vi "dispense test.vi"() -> ()   [LabVIEW 2021]
uses:
  Classes/Controller/Controller.lvclass
  Classes/Controller/Dispenser/Dispenser.lvclass
panel:
  out "current time 3":timestamp
  out "current time 2":timestamp
  out "current time":timestamp
  out "Adjusted Dispensing Time (ms)":dbl
  out "Start time":timestamp
  out "end time":timestamp
  out "Iteration":i32
  in  "Time (ms)":dbl
  out "Dispense on":bool
  out "error out":errorcluster
  in  "error in (no error)":errorcluster
  in  "Pressure (psi)":i16=20
  in  "Dispense":bool
  in  "stop":bool
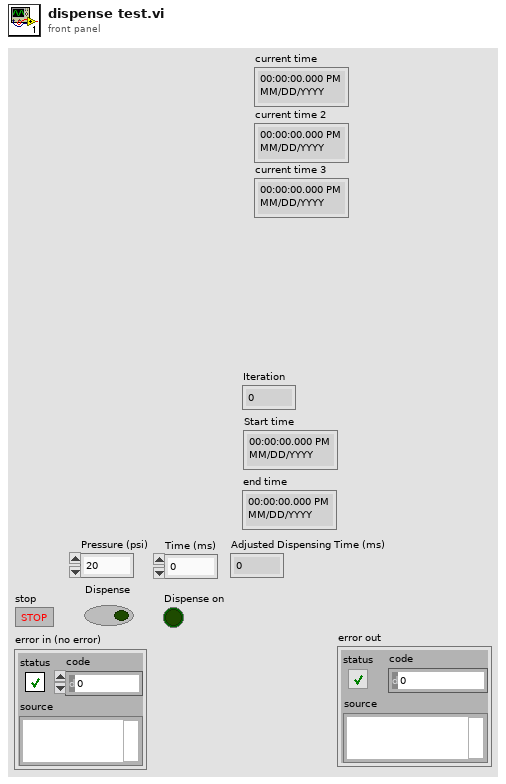
[diagram p1: front panel]
types:
  T1 = typedef "Controller.lvclass/Controllers.ctl" = cluster{"I-O.lvclass":refnum<class "I-O.lvclass">, "Gantry":refnum<k24>, "Dispenser":refnum<visa-resource-name>}
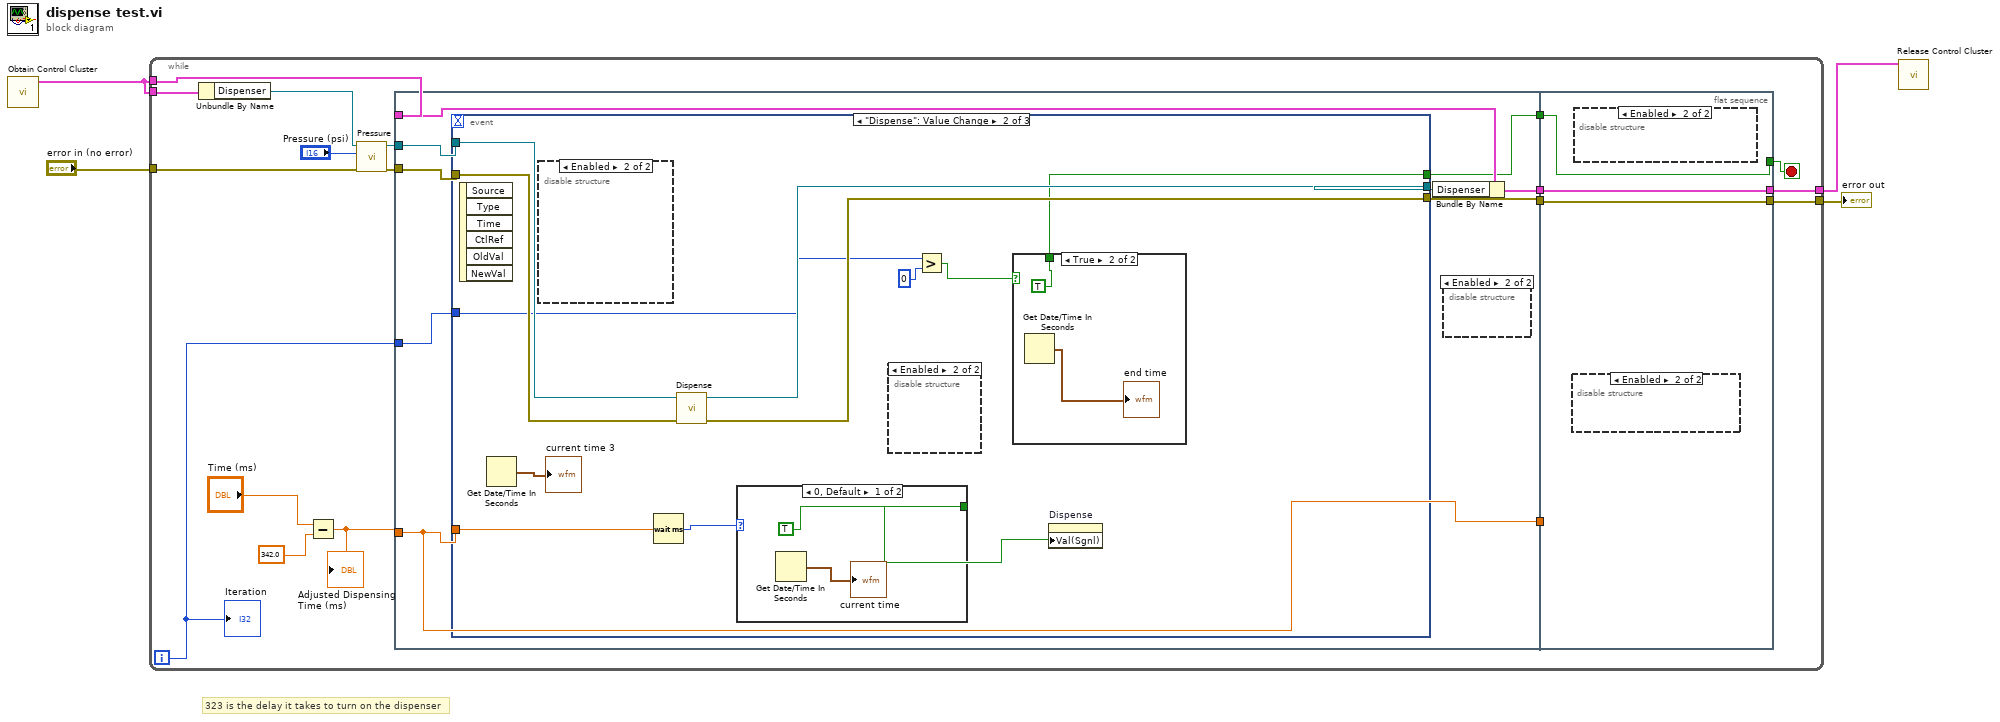
[diagram p0: block diagram]
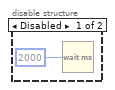
[diagram p2: hidden frame]
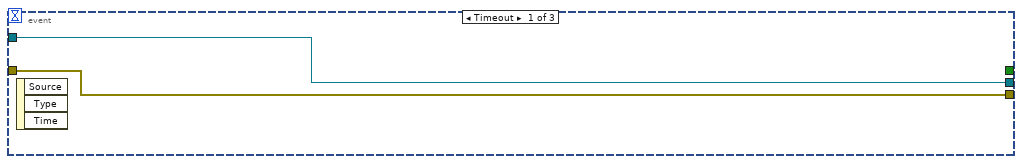
[diagram p3: hidden frame]
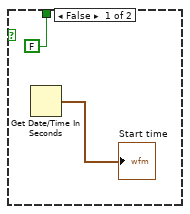
[diagram p4: hidden frame]
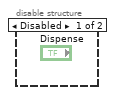
[diagram p5: hidden frame]
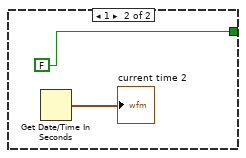
[diagram p6: hidden frame]
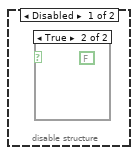
[diagram p7: hidden frame]
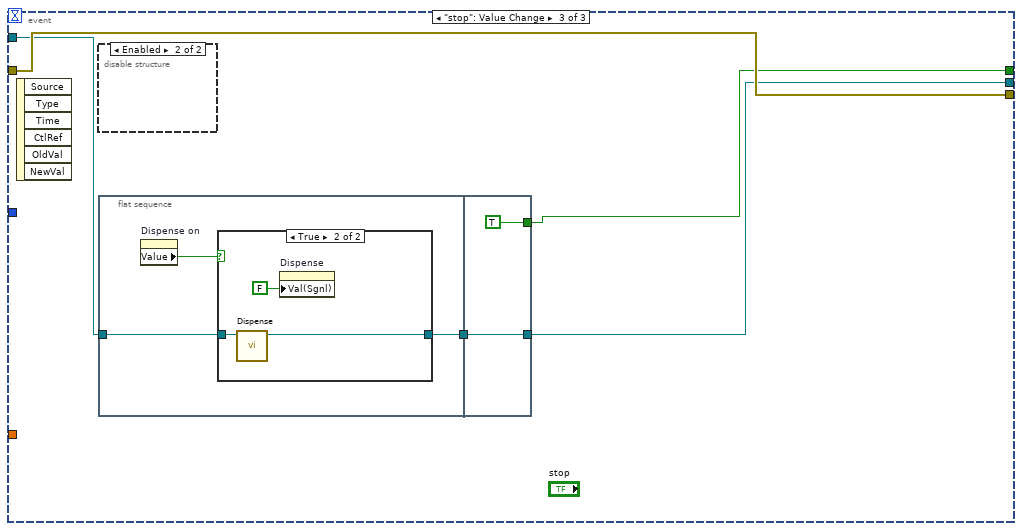
[diagram p9: hidden frame]
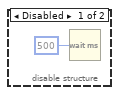
[diagram p10: hidden frame]
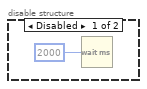
[diagram p12: hidden frame]
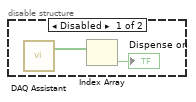
[diagram p13: hidden frame]
diagram:
  # "323 is the delay it takes to turn on the dispenser"
  n1 = call "Obtain Control Cluster.vi"() -> ("Control Out"=w3:T1)  [unwired: 11 in]
  n2 = while {
    tunnel: w3 -> [w22]
    tunnel: "error in (no error)" -> [w19]
    tunnel: w3 -> [w17]
    tunnel: [w16] -> w2
    tunnel: [w14] -> w1
    i -> [w8]
    stop <- w13 stop-if-true
    n3 = Unbundle By Name(w22) -> ("Dispenser"=w21:refnum<visa-resource-name>)
    n4 = Subtract(x="Time (ms)", y=342.0) -> (x-y=w5:dbl)
    "Adjusted Dispensing Time (ms)" <- w5
    n5 = call "Pressure.vi"("error in (no error)"=w19, "Pressure"="Pressure (psi)", "VISA resource name"=w21) -> ("error out"=w15:errorcluster, "VISA resource name out"=w18:refnum<visa-resource-name>)  [unwired: 7 in]
    n6 = flat-sequence {
      tunnel: w18 -> [w31]
      tunnel: w17 -> [w30]
      tunnel: w15 -> [w28]
      tunnel: [w29] -> w12
      tunnel: [w27] -> w11
      tunnel: [w26] -> w10
      tunnel: w5 -> [w24]
      tunnel: [w24] -> w9
      tunnel: w8 -> [w23]
      tunnel: [w70] -> w13
      tunnel: [w71] -> w14
      tunnel: [w72] -> w16
      tunnel: w12 -> [w72]
      tunnel: w11 -> [w71]
      tunnel: w10 -> [w70]
      tunnel: w9 -> [_]
      frame #0 {
        n7 = event shown="[1] \"Dispense\": Value Change" {
          selector: _ -> [_ _ _]
          dyn-events: _ -> [_ _ _]
          timeout: _ -> [_ _ _]
          tunnel: w31 -> [w34 w46 w59]
          tunnel: [w34 w45 w58] -> w25
          tunnel: w28 -> [w33 w44 w60]
          tunnel: [w33 w43 w60] -> w27
          tunnel: [_ w38 w56] -> w26
          tunnel: w24 -> [_ w42 _]
          tunnel: w23 -> [_ w37 _]
          event Timeout {
            n8 = event-data() -> ()  [unwired: 1 in, 3 out]
          }
          event "Dispense": Value Change {
            n9 = event-data() -> ()  [unwired: 1 in, 6 out]
            n10 = Get Date/Time In Seconds() -> (seconds since 1Jan1904=→"current time 3":timestamp)
            n11 = disable-structure shown="Enabled" {
              frame Disabled {
                n12 = case shown="True" {
                  selector: _ -> [_ _]
                  frame False {
                  }
                  frame True {
                    w55 = FALSE
                  }
                }
              }
              frame Enabled {
              }
            }
            n13 = Wait (ms)(milliseconds to wait=w42) -> (millisecond timer value=w41:u32)
            n14 = call "Dispense.vi"("error in (no error)"=w44, "Dispenser In"=w46) -> ("error out"=w43:errorcluster, "Dispenser Out"=w45:refnum<visa-resource-name>)  [unwired: 8 in]
            n15 = case shown="0, Default" w41 {
              tunnel: [TRUE FALSE] -> w40
              frame 0, Default {
                n16 = Get Date/Time In Seconds() -> (seconds since 1Jan1904=→"current time":timestamp)
              }
              frame 1 {
                n17 = Get Date/Time In Seconds() -> (seconds since 1Jan1904=→"current time 2":timestamp)
              }
            }
            n18 = disable-structure shown="Enabled" {
              frame Disabled {
              }
              frame Enabled {
              }
            }
            n19 = Greater?(x=w37, y=0) -> (0:w36:bool)
            n20 = case shown="True" w36 {
              tunnel: [FALSE TRUE] -> w38
              frame False {
                n21 = Get Date/Time In Seconds() -> (seconds since 1Jan1904=→"Start time":timestamp)
              }
              frame True {
                n22 = Get Date/Time In Seconds() -> (seconds since 1Jan1904=→"end time":timestamp)
              }
            }
            n23 = property on="Dispense" class="Bool (strict)"("Val(Sgnl)"=w40) -> ()  [unwired: 2 in, 2 out]
          }
          event "stop": Value Change {
            n24 = event-data() -> ()  [unwired: 1 in, 6 out]
            n25 = disable-structure shown="Enabled" {
              frame Disabled {
                n26 = Wait (ms)(milliseconds to wait=u32 500) -> ()  [unwired: 1 out]
              }
              frame Enabled {
              }
            }
            n27 = flat-sequence {
              tunnel: w59 -> [w64]
              tunnel: [w63] -> w57
              tunnel: [w69] -> w58
              tunnel: w57 -> [w69]
              tunnel: [TRUE] -> w56
              frame #0 {
                n28 = property on="Dispense on" class="Bool (strict)"() -> ("Value"=w62:bool)  [unwired: 2 in, 2 out]
                n29 = case shown="True" w62 {
                  tunnel: w64 -> [_ w67]
                  tunnel: [_ w66] -> w63
                  frame False {
                  }
                  frame True {
                    n30 = call "Dispense.vi"("Dispenser In"=w67) -> ("Dispenser Out"=w66:refnum<visa-resource-name>)  [unwired: 9 in, 1 out]
                    n31 = property on="Dispense" class="Bool (strict)"("Val(Sgnl)"=FALSE) -> ()  [unwired: 2 in, 2 out]
                  }
                }
              }
              frame #1 {
              }
            }
          }
        }
        n32 = Bundle By Name(cluster=w30, "Dispenser"=w25) -> (w29:T1)
        n33 = disable-structure shown="Enabled" {
          frame Disabled {
            n34 = Wait (ms)(milliseconds to wait=u32 2000) -> ()  [unwired: 1 out]
          }
          frame Enabled {
          }
        }
      }
      frame #1 {
        n35 = disable-structure shown="Enabled" {
          frame Disabled {
            n36 = Wait (ms)(milliseconds to wait=u32 2000) -> ()  [unwired: 1 out]
          }
          frame Enabled {
          }
        }
        n37 = disable-structure shown="Enabled" {
          frame Disabled {
            n38 = call "DAQ Assistant"() -> ("data"=w75:bool[])  [unwired: 17 in, 2 out]
            n39 = Index Array(array=w75) -> (element=→"Dispense on":bool)  [unwired: 1 in]
          }
          frame Enabled {
          }
        }
      }
    }
    "Iteration" <- w8
  }
  "error out" <- w1
  n40 = call "Release Control Cluster.vi"("output cluster"=w2) -> ()  [unwired: 11 in]
